vi "CRYCalc Peak Detection.vi"(8 "Loose Particle dT":dbl, 9 "Loose part Info":T1, 10 "Fs":dbl=44100.0 min=1.0, 11 "Loose Particle Envelope In":dbl[](array[numeric])) -> (0 "number of peaks":i32, 3 "Loose Particle Threshold":dbl[](array[numeric]))   [LabVIEW 2013]
uses:
  <vilib>/Analysis/1siggen.llb/Ramp Pattern by Samples.vi
  <vilib>/addons/Wavelet Analysis/application.llb/WA Multiscale Peak Detection (Array).vi
  <vilib>/Analysis/NI_AALBase.lvlib
  <vilib>/addons/_Advanced Signal Processing/NI_AdvSigProcWA.lvlib
panel:
  out "Array 3":i32[](array[numeric])
  out "Array 2":i32[](array[numeric])
  out "Array":i32[](array[numeric])
  out "number of peaks 2":i32
  in  "width(Min Samples)":i32=8
  out "number of valleys":i32
  out "peak plot":cluster{"Locations":dbl[], "Amplitudes":dbl[]}[](graph)
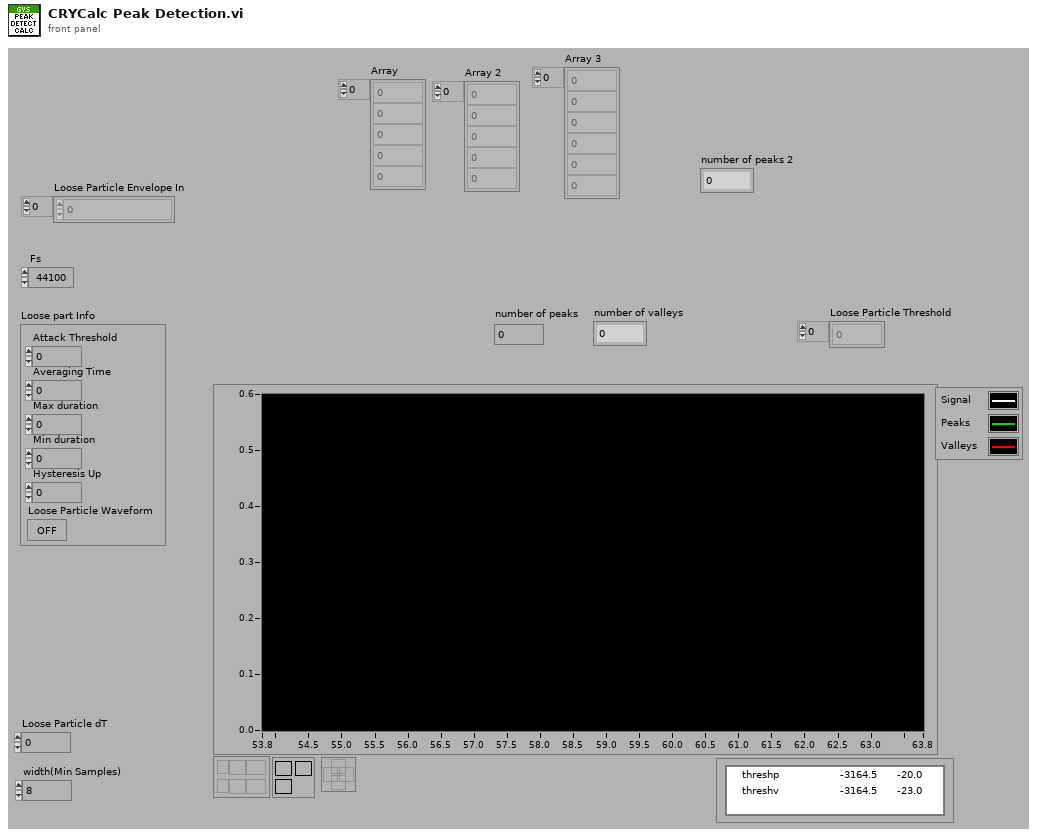
[diagram p1: front panel]
types:
  T1 = cluster{"Attack Threshold":dbl, "Averaging Time":dbl, "Max duration":dbl, "Min duration":dbl, "Hysteresis Up":dbl, "Loose Particle Waveform":bool}
  T2 = cluster{"Ramp Pattern":dbl[], "Loose Particle Envelope In":dbl[]}
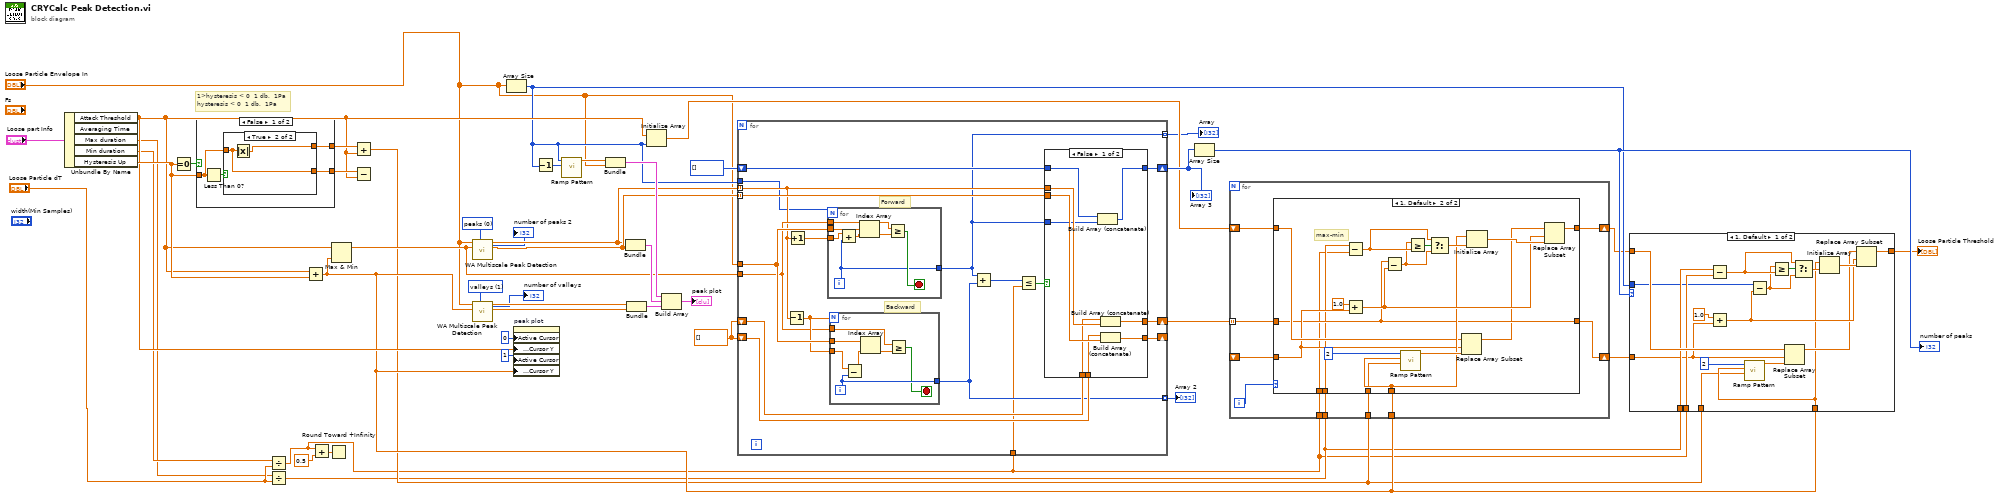
[diagram p0: block diagram]
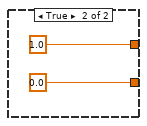
[diagram p5: hidden frame]
diagram:
  w24 = dbl[] []
  w34 = u16 0 items=["peaks", "valleys"] ("peaks/valleys")
  w35 = u16 1 items=["peaks", "valleys"] ("peaks/valleys")
  # "1>hysteresis < 0  1 db,  1Pa\nhysteresis < 0  1 db,  1Pa"
  n1 = Unbundle By Name("Loose part Info") -> ("Attack Threshold"=w27:dbl, "Max duration"=w5:dbl, "Min duration"=w6:dbl, "Hysteresis Up"=w28:dbl)  [unwired: 1 out]
  n2 = Equal To 0?(x=w28) -> (x = 0?=w32:bool)
  n3 = case shown="False" w32 {
    tunnel: [w47 1.0 ("level")] -> w31
    tunnel: [w46 0.0 ("level")] -> w30
    tunnel: w28 -> [w48 _]
    frame False {
      n4 = Less Than 0?(x=w48) -> (x < 0?=w49:bool)
      n5 = case shown="True" w49 {
        tunnel: w48 -> [w50 w51]
        tunnel: [w50 w52] -> w47
        tunnel: [w50 w51] -> w46
        frame False {
        }
        frame True {
          n6 = Absolute Value(x=w51) -> (abs(x)=w52:dbl)
        }
      }
    }
    frame True {
    }
  }
  n7 = Divide(x=w6, y="Loose Particle dT") -> (x/y=w1:dbl)
  n8 = Divide(x=w5, y="Loose Particle dT") -> (x/y=w2:dbl)
  n9 = Add(x=w27, y=w28) -> (x+y=w14:dbl)
  n10 = Add(x=w1, y=0.5) -> (x+y=w3:dbl)
  n11 = Round Toward +Infinity(x=w3) -> ()  [unwired: 1 out]
  n12 = Max & Min(x=w27, y=w14) -> (max(x,y)=w21:dbl)  [unwired: 1 out]
  n13 = Add(x=w31, y=w27) -> (x+y=w13:dbl)
  n14 = Subtract(x=w30, y=w27) -> ()  [unwired: 1 out]
  n15 = call-poly <vilib>:"WA Multiscale Peak Detection.vi"("peaks/valleys"=w34, "threshold"=w21, "signal"="Loose Particle Envelope In") -> ("amplitude"=w26:dbl[], "location"=w25:dbl[], "number of peaks"=→"number of peaks 2":i32)  [unwired: 4 in, 2 out]
  n16 = call-poly <vilib>:"WA Multiscale Peak Detection.vi"("peaks/valleys"=w35, "threshold"=w14, "signal"="Loose Particle Envelope In") -> ("amplitude"=w38:dbl[], "location"=w39:dbl[], "number of peaks"=→"number of valleys":i32)  [unwired: 4 in, 2 out]
  n17 = Array Size(array="Loose Particle Envelope In") -> (size(s)=w16:i32)
  n18 = property on="peak plot" class="XYGraph (strict)"("Active Cursor"=u32 0, "Cursor.Cursor Position:Cursor Y"=w27, "Active Cursor"=u32 1, "Cursor.Cursor Position:Cursor Y"=w14) -> ()  [unwired: 2 in, 2 out]
  n19 = Decrement(x=w16) -> (x-1=w44:i32)
  n20 = call-poly <vilib>:"Ramp Pattern.vi"("end"=w44, "samples"=w16) -> ("Ramp Pattern"=w45:dbl[])  [unwired: 8 in, 1 out]
  n21 = Bundle("Ramp Pattern"=w45, "Loose Particle Envelope In"="Loose Particle Envelope In") -> (w43:T2)  [unwired: 1 in]
  n22 = Bundle("location"=w25, "amplitude"=w26) -> (w33:cluster{"location":dbl[], "amplitude":dbl[]})  [unwired: 1 in]
  n23 = Bundle("location"=w39, "amplitude"=w38) -> (w37:cluster{"location":dbl[], "amplitude":dbl[]})  [unwired: 1 in]
  n24 = Initialize Array(w27, w16) -> (w19:dbl[])
  n25 = Build Array(w43, w33, w37) -> (→"peak plot":cluster{"location":dbl[], "amplitude":dbl[]}[])
  n26 = for {
    tunnel: w25 -> [w60] mode=indexing
    tunnel: w26 -> [w67] mode=indexing
    tunnel: w21 -> [w69]
    tunnel: "Loose Particle Envelope In" -> [w71]
    tunnel: w16 -> [w59]
    shift-right: [w66] -> w23
    shift-left: w24 -> [w64]
    shift-right: [w65] -> _
    shift-left: w24 -> [w63]
    shift-right: [w62] -> w20
    shift-left: i32[] [] ("Array 2") -> [w61]
    tunnel: [w57] -> w9 mode=indexing
    tunnel: [w58] -> w8 mode=indexing
    tunnel: w1 -> [w56]
    # "Backward"
    # "Forward"
    n27 = Decrement(x=w60) -> (x-1=w70:dbl)
    n28 = Increment(x=w60) -> (x+1=w72:dbl)
    n29 = for {
      N: w59 -> [_]
      tunnel: w72 -> [w97]
      tunnel: w71 -> [w98]
      tunnel: w69 -> [w95]
      tunnel: [w92] -> w57
      i -> [w92]
      stop <- w93 stop-if-true
      n30 = Add(x=w97, y=w92) -> (x+y=w96:dbl)
      n31 = Index Array(array=w98, index=w96) -> (element=w94:dbl)
      n32 = Greater Or Equal?(x=w95, y=w94) -> (x >= y?=w93:bool)
    }
    n33 = for {
      N: w70 -> [_]
      tunnel: w70 -> [w90]
      tunnel: w71 -> [w91]
      tunnel: w69 -> [w88]
      tunnel: [w86] -> w58
      i -> [w86]
      stop <- w85 stop-if-true
      n34 = Subtract(x=w90, y=w86) -> (x-y=w89:dbl)
      n35 = Index Array(array=w91, index=w89) -> (element=w87:dbl)
      n36 = Greater Or Equal?(x=w88, y=w87) -> (x >= y?=w85:bool)
    }
    n37 = Add(x=w57, y=w58) -> (x+y=w55:i32)
    n38 = Less Or Equal?(x=w55, y=w56) -> (x <= y?=w68:bool)
    n39 = case shown="False" w68 {
      tunnel: w67 -> [w79 _]
      tunnel: w60 -> [w78 _]
      tunnel: w57 -> [w73 _]
      tunnel: [w80 w83] -> w65
      tunnel: [w81 w84] -> w66
      tunnel: w64 -> [w77 w84]
      tunnel: w63 -> [w76 w83]
      tunnel: [w75 w82] -> w62
      tunnel: w61 -> [w74 w82]
      frame False {
        n40 = Build Array (concatenate)(w74, w73) -> (w75:i32[])
        n41 = Build Array (concatenate)(w77, w78) -> (w81:dbl[])
        n42 = Build Array (concatenate)(w76, w79) -> (w80:dbl[])
      }
      frame True {
      }
    }
  }
  "Array" <- w9
  "Array 2" <- w8
  "Array 3" <- w20
  n43 = Array Size(array=w20) -> (size(s)=w18:i32)
  "number of peaks" <- w18
  n44 = for {
    tunnel: w23 -> [w99] mode=indexing
    tunnel: w14 -> [w108]
    shift-right: [w107] -> w15
    shift-left: w19 -> [w102]
    shift-right: [w105] -> w17
    shift-left: _ -> [w104]
    tunnel: w13 -> [w103]
    tunnel: w2 -> [w101]
    tunnel: w1 -> [w100]
    i -> [w106]
    n45 = case shown="1, Default" w106 {
      tunnel: w102 -> [w110 w119]
      tunnel: w99 -> [w109 w117]
      tunnel: w108 -> [_ w121]
      tunnel: [w110 w111] -> w107
      tunnel: [w109 w117] -> w105
      tunnel: w104 -> [_ w118]
      tunnel: w103 -> [_ w120]
      tunnel: w101 -> [_ w116]
      tunnel: w100 -> [_ w115]
      frame 0 {
      }
      frame 1, Default {
        # "max-min"
        n46 = Subtract(x=w116, y=w115) -> (x-y=w126:dbl)
        n47 = Add(x=1.0, y=w118) -> (x+y=w123:dbl)
        n48 = Subtract(x=w117, y=w123) -> (x-y=w125:dbl)
        n49 = call-poly <vilib>:"Ramp Pattern.vi"("start"=w120, "end"=w121, "samples"=2) -> ("Ramp Pattern"=w122:dbl[])  [unwired: 7 in, 1 out]
        n50 = Greater Or Equal?(x=w125, y=w126) -> (x >= y?=w127:bool)
        n51 = Select(t=w126, s=w127, f=w125) -> (s? t:f=w124:dbl)
        n52 = Replace Array Subset(array=w119, new element=w122, index=w118) -> (w114:dbl[])
        n53 = Initialize Array(w121, w124) -> (w128:dbl[])
        n54 = Replace Array Subset(array=w114, new element=w128, index=w123) -> (w111:dbl[])
      }
    }
  }
  n55 = case shown="1, Default" w18 {
    tunnel: w17 -> [w131 _]
    tunnel: w16 -> [w135 _]
    tunnel: w15 -> [w138 w147]
    tunnel: w1 -> [w137 _]
    tunnel: w2 -> [w136 _]
    tunnel: w14 -> [w134 _]
    tunnel: w13 -> [w133 _]
    tunnel: [w132 w147] -> w12
    frame 1, Default {
      n56 = Subtract(x=w136, y=w137) -> (x-y=w144:dbl)
      n57 = Add(x=1.0, y=w131) -> (x+y=w141:dbl)
      n58 = call-poly <vilib>:"Ramp Pattern.vi"("start"=w133, "end"=w134, "samples"=2) -> ("Ramp Pattern"=w140:dbl[])  [unwired: 7 in, 1 out]
      n59 = Subtract(x=w135, y=w141) -> (x-y=w143:dbl)
      n60 = Greater Or Equal?(x=w143, y=w144) -> (x >= y?=w145:bool)
      n61 = Replace Array Subset(array=w138, new element=w140, index=w131) -> (w139:dbl[])
      n62 = Select(t=w144, s=w145, f=w143) -> (s? t:f=w142:dbl)
      n63 = Initialize Array(w134, w142) -> (w146:dbl[])
      n64 = Replace Array Subset(array=w139, new element=w146, index=w141) -> (w132:dbl[])
    }
    frame 0 {
    }
  }
  "Loose Particle Threshold" <- w12
